vi "Draw_Block.vi"(8 "Block":T1 {"orientaion" items=["up", "down", "left", "right"]; "type" items=["t", "rl", "ll", "rz", "lz", "square", "line"]}, 11 "Input Array":bool[][](array[boolean])) -> (3 "Output Array":bool[][](array[boolean]))   [LabVIEW 2015]
uses:
  block.ctl
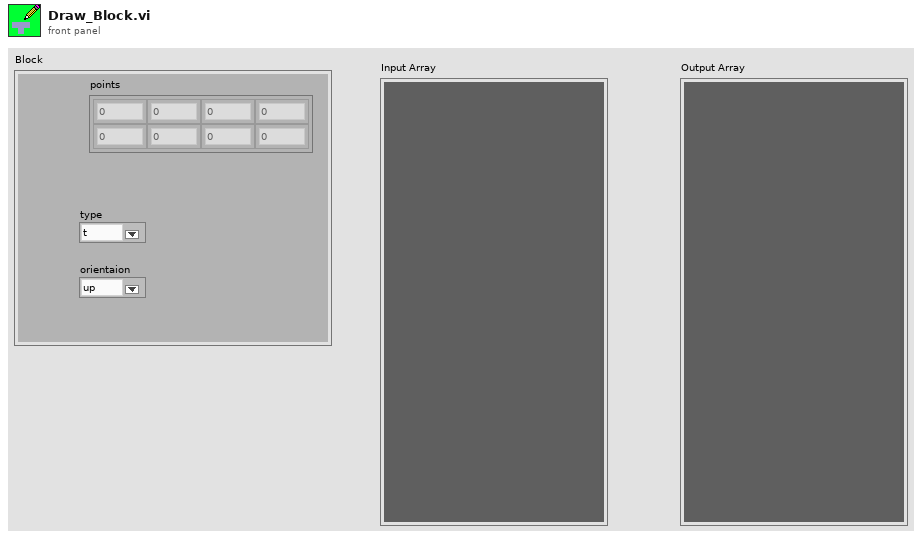
[diagram p1: front panel]
types:
  T1 = typedef "block.ctl" = cluster{"points":dbl[][], "type":u16, "orientaion":u16}
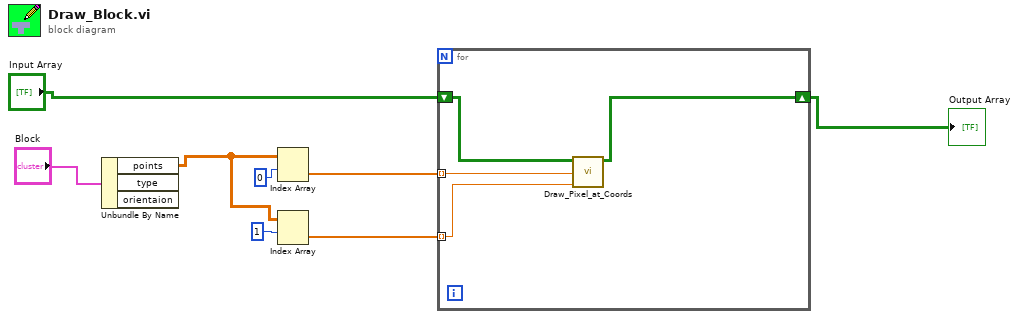
[diagram p0: block diagram]
diagram:
  n1 = Unbundle By Name("Block") -> ("points"=w5:dbl[][])  [unwired: 2 out]
  n2 = Index Array(array=w5, index (row)=0) -> (element=w4:dbl[])  [unwired: 1 in]
  n3 = Index Array(array=w5, index (row)=1) -> (element=w3:dbl[])  [unwired: 1 in]
  n4 = for {
    tunnel: w4 -> [w12] mode=indexing
    tunnel: w3 -> [w11] mode=indexing
    shift-right: [w10] -> w1
    shift-left: "Input Array" -> [w9]
    n5 = call "Draw_Pixel_at_Coords.vi"("y-axis 2"=w11, "x-axis"=w12, "Input array"=w9) -> ("Ouput array"=w10:bool[][])  [unwired: 8 in]
  }
  "Output Array" <- w1
